vi "Handle Error.vi"(8 "error in (no error)":errorcluster, 11 "Actor_Autotest in":refnum<class "Actor_Autotest.lvclass">) -> (0 "error out":errorcluster, 2 "stop actor?":bool=TRUE, 3 "Actor_Autotest out":refnum<class "Actor_Autotest.lvclass">)   [LabVIEW 2020, in "Library Core.lvlib" / "Actor_Autotest.lvlib" / "Actor_Autotest.lvclass"]
doc: "(<B>Filename</B>: Actor Framework.lvlib:Actor.lvclass:Handle Error.vi)\n\nDefines how the actor handles an error that occurred while processing a message. By default, this method does nothing except stop the actor."
uses:
  Actor_Autotest.lvclass
  <vilib>/ActorFramework/Actor/Actor.lvclass
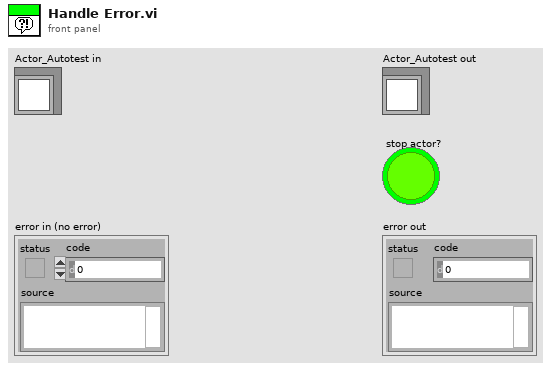
[diagram p1: front panel]
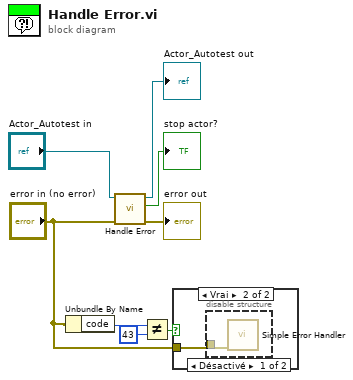
[diagram p0: block diagram]
diagram:
  n1 = Unbundle By Name("error in (no error)") -> ("code"=w2:i32)
  n2 = call-parent "Handle Error.vi"("error in (no error)"="error in (no error)", "Actor in"="Actor_Autotest in") -> ("error out"=→"error out":errorcluster, "stop actor?"=→"stop actor?":bool, "Actor out"=→"Actor_Autotest out":refnum<class "Actor_Autotest.lvclass">)  [unwired: 7 in]
  n3 = Not Equal?(x=w2, y=43) -> (x != y?=w3:bool)
  n4 = case shown="Vrai" w3 {
    tunnel: "error in (no error)" -> [_ w9]
    frame False {
    }
    frame True {
      n5 = disable-structure shown="Désactivé" {
        disable-tunnel: w9 -> [w10 _]
        frame Disabled {
          n6 = call <vilib>:"Simple Error Handler.vi"("error in (no error)"=w10) -> ()  [unwired: 4 in, 5 out]
        }
        frame Enabled {
        }
      }
    }
  }
